vi "Read Color.vi"(8 "error in (no error)":errorcluster, 11 "RectangleShape in":refnum<class "RectangleShape.lvclass">) -> (0 "error out":errorcluster, 2 "Color out":u32(colorbox), 3 "RectangleShape out":refnum<class "RectangleShape.lvclass">)   [LabVIEW 2022 SP3, in "RectangleShape.lvclass"]
uses:
  RectangleShape.lvclass
  RectangleShape.lvclass/RectangleShape.ctl
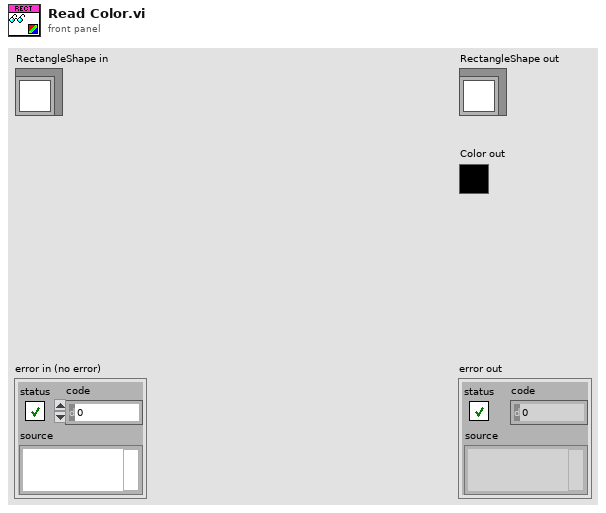
[diagram p1: front panel]
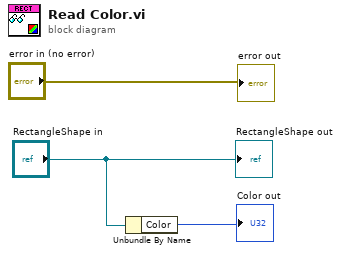
[diagram p0: block diagram]
diagram:
  n1 = Unbundle By Name("RectangleShape in") -> ("Color"=→"Color out":u32)
  "error out" <- "error in (no error)"
  "RectangleShape out" <- "RectangleShape in"
